vi "Get dBm Impedance.vi"(8 "error in (no error)":errorcluster, 11 "VISA resource name":refnum<visa-resource-name>) -> (0 "error out":errorcluster, 2 "dBm Impedance":i32, 3 "VISA resource name out":refnum<visa-resource-name>)   [LabVIEW 2014, in "Fluke 5XXX Series Multicalibrators.lvlib"]
doc: "This VI gets the impedance used for dBm outputs (ac volts).\n\nNote:\n\nThis VI is available only for instrument model 5520A."
uses:
  Fluke 5XXX Series Multicalibrators.lvlib
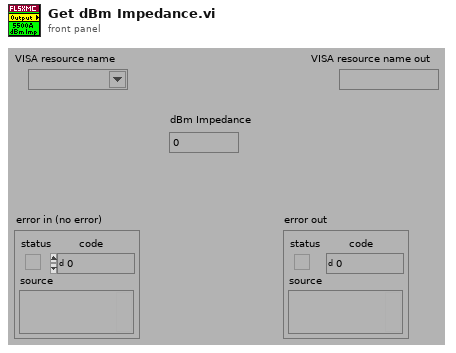
[diagram p1: front panel]
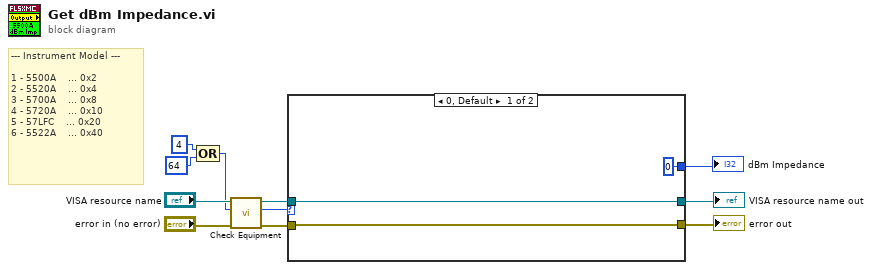
[diagram p0: block diagram]
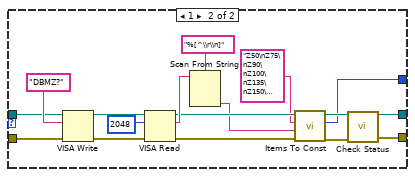
[diagram p2: hidden frame]
diagram:
  # "--- Instrument Model ---\n\n1 - 5500A    ... 0x2\n2 - 5520A    ... 0x4\n3 - 5700A    ... 0x8\n4 - 5720A    ... 0x10\n5 - 57LFC    ... 0x20\n6 - 5522A    ... 0x40"
  n1 = Compound Arithmetic op=OR(4 ("Numeric"), 64 ("Numeric")) -> (w1:i32)
  n2 = call "Check Equipment.vi"("error in (no error)"="error in (no error)", "Bit Mask"=w1, "VISA resource name"="VISA resource name") -> ("error out"=w11:errorcluster, "Present?"=w10:u32, "VISA resource name out"=w9:refnum<visa-resource-name>)  [unwired: 6 in]
  n3 = case shown="0, Default" w10 {
    tunnel: [w13 w23] -> w5
    tunnel: w11 -> [w14 w25]
    tunnel: w9 -> [w13 w24]
    tunnel: [w14 w22] -> w8
    tunnel: [0 ("Index") w17] -> w4
    frame 0, Default {
    }
    frame 1 {
      n4 = VISA Write(VISA resource name=w24, write buffer="DBMZ?", error in (no error)=w25) -> (VISA resource name out=w30:refnum<visa-resource-name>, error out=w29:errorcluster)  [unwired: 1 out]
      n5 = VISA Read(VISA resource name=w30, byte count=u32 2048 ("byte count (0)"), error in (no error)=w29) -> (VISA resource name out=w19:refnum<visa-resource-name>, read buffer=w26:string, error out=w20:errorcluster)  [unwired: 1 out]
      n6 = Scan From String(format string="%[^\\r\\n]", input string=w26) -> (output 1=w15:string)  [unwired: 3 in, 3 out]
      n7 = call "Items To Const.vi"("error in (no error)"=w20, "String Item"=w15, "Multi-Line String"="Z50\nZ75\nZ90\nZ100\nZ135\nZ150\nZ300\nZ600\nZ900\nZ1000\nZ1200", "VISA resource name"=w19) -> ("error out"=w21:errorcluster, "Index"=w17:i32, "VISA resource name out"=w18:refnum<visa-resource-name>)  [unwired: 5 in]
      n8 = call "Check Status.vi"("VISA resource name"=w18, "error in (no error)"=w21) -> ("VISA resource name out"=w23:refnum<visa-resource-name>, "error out"=w22:errorcluster)  [unwired: 12 in]
    }
  }
  "dBm Impedance" <- w4
  "VISA resource name out" <- w5
  "error out" <- w8
